vi "WS1050 Read From Configuration File.vi"(8 "error in (no error)":errorcluster, 11 "Configuration File Path":path=path "S:/Software_Control/RELEASED_SOFTWARE_RUN_ALL_TEST_FROM_HERE/PACKAGE/TMN/TMN1P5-Test-System/WS1050_vsa20-20_Temp.txt") -> (0 "error out":errorcluster, 3 "Configuration":T1)   [LabVIEW 2017]
uses:
  Andy's LLB LV2012/Read_Test_Limits/TSTR Configuration Cluster1.0.ctl
  <vilib>/Utility/config.llb/Read Key (String).vi
  <vilib>/Utility/config.llb/NI_LVConfig.lvlib
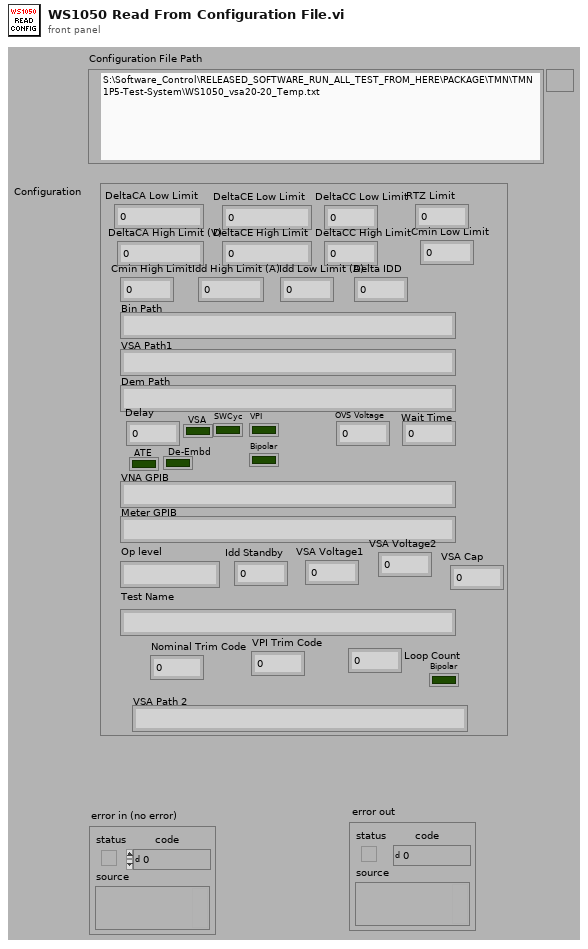
[diagram p1: front panel]
types:
  T1 = typedef "TSTR Configuration Cluster1.0.ctl" = cluster{"DeltaCA Low Limit ":dbl, "DeltaCA High Limit (V)":dbl, "DeltaCE Low Limit ":dbl, "DeltaCE High Limit":dbl, "DeltaCC Low Limit":dbl, "DeltaCC High Limit":dbl, "RTZ Limit":dbl, "Cmin Low Limit":dbl, "Cmin High Limit":dbl, "Idd High Limit (A)":dbl, "Idd Low Limit (A)":dbl, "Delta IDD":dbl, "Bin Path":string, "VSA Path1":string, "Dem Path":string, "Delay":dbl, "VSA":bool, "SWCyc":bool, "VPI":bool, "Bipolar":bool, "OVS Voltage":dbl, "Wait Time":dbl, "ATE":bool, "VNA GPIB":string, "Meter GPIB ":string, "Op level":string, "Idd Standby":dbl, "VSA Voltage1":dbl, "VSA Cap":dbl, "Test Name":string, "Nominal Trim Code":i32, "VPI Trim Code":i32, "De-Embd":bool, "Loop Count":i32, "Bipolar":bool, "VSA Path 2":string, "VSA Voltage2":dbl}
  T2 = typedef "NI_LVConfig.lvlib/Config Data RefNum.ctl" = refnum<k1>
  T3 = cluster{dbl, dbl, dbl, dbl, dbl, dbl, dbl, dbl, dbl, dbl, dbl, dbl, "value":string, "value":string, "value":string, dbl, bool, bool, bool, bool, dbl, dbl, bool, "value":string, "value":string, "value":string, dbl, dbl, dbl, "value":string, i32, i32, bool, i32, bool, "value":string, dbl}
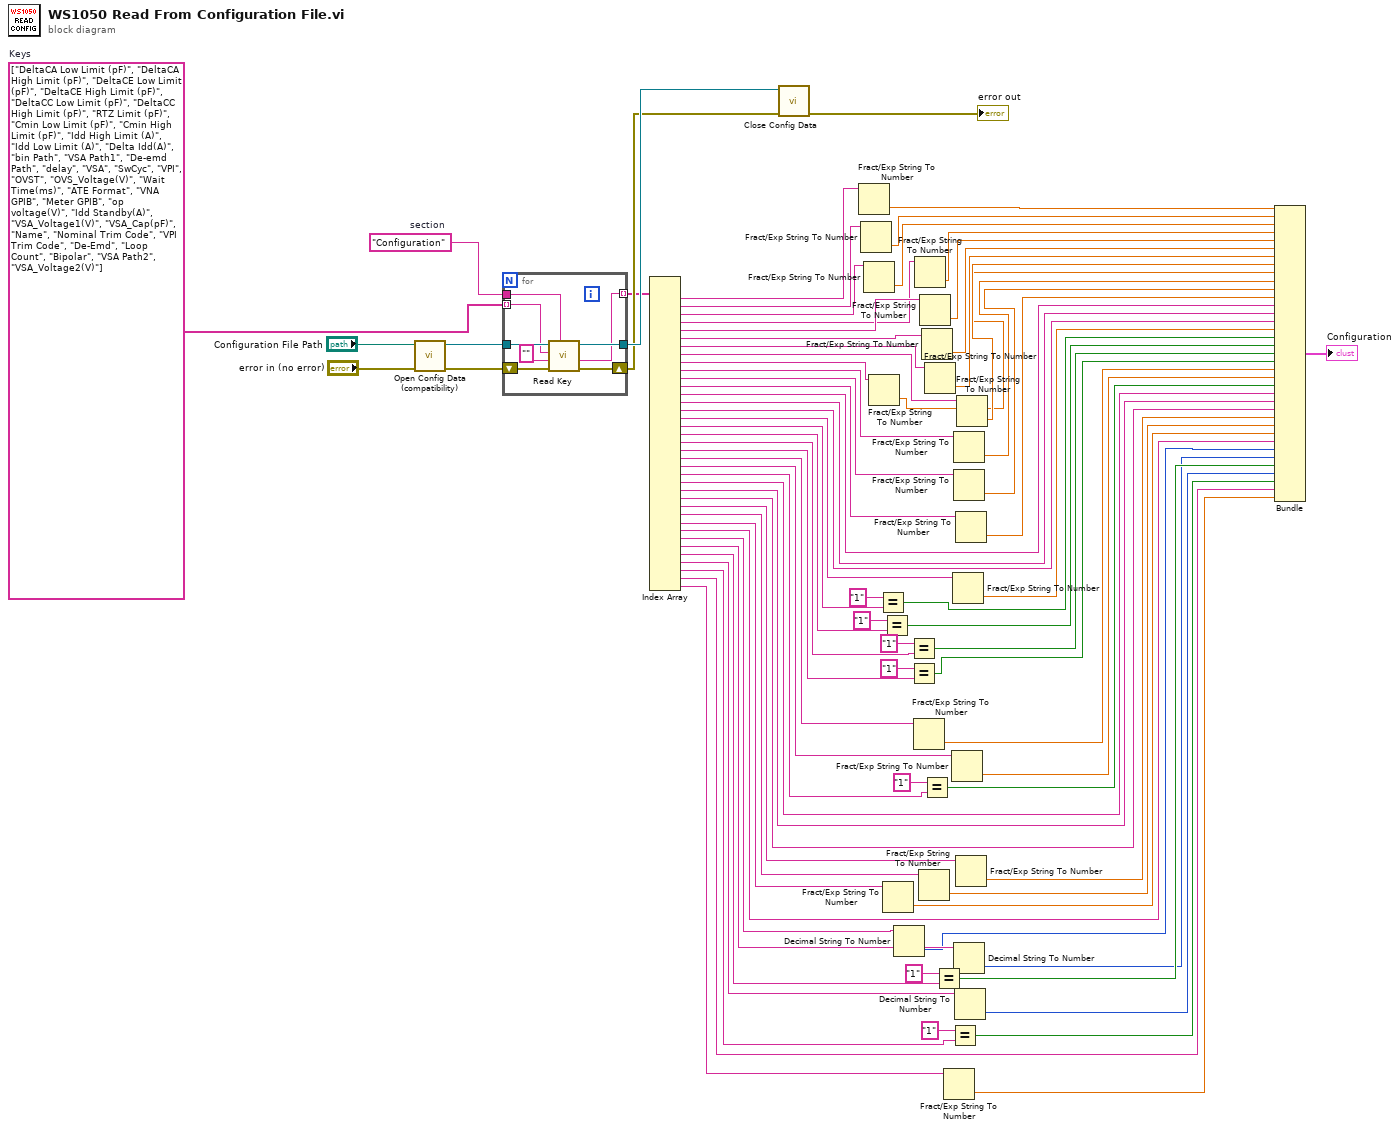
[diagram p0: block diagram]
diagram:
  w78 = string[] ["DeltaCA Low Limit (pF)", "DeltaCA High Limit (pF)", "DeltaCE Low Limit (pF)", "DeltaCE High Limit (pF)", "DeltaCC Low Limit (pF)", "DeltaCC High Limit (pF)", "RTZ Limit (pF)", "Cmin Low Limit (pF)", "Cmin High Limit (pF)", "Idd High Limit (A)", "Idd Low Limit (A)", "Delta Idd(A)", "bin Path", "VSA Path1", "De-emd Path", "delay", "VSA", "SwCyc", "VPI", "OVST", "OVS_Voltage(V)", "Wait Time(ms)", "ATE Format", "VNA GPIB", "Meter GPIB", "op voltage(V)", "Idd Standby(A)", "VSA_Voltage1(V)", "VSA_Cap(pF)", "Name", "Nominal Trim Code", "VPI Trim Code", "De-Emd", "Loop Count", "Bipolar", "VSA Path2", "VSA_Voltage2(V)"]  # Keys
  w79 = "Configuration"  # section
  n1 = call <vilib>:"Open Config Data (compatibility).vi"("error in (no error)"="error in (no error)", "configuration file path"="Configuration File Path") -> ("error out"=w82:errorcluster, "refnum"=w84:T2)  [unwired: 7 in, 1 out]
  n2 = for {
    tunnel: w84 -> [w92]
    tunnel: [w91] -> w83
    tunnel: w79 -> [w88]
    tunnel: [w87] -> w77 mode=indexing
    shift-right: [w89] -> w81
    shift-left: w82 -> [w90]
    tunnel: w78 -> [w86] mode=indexing
    n3 = call-poly <vilib>:"Read Key.vi"("section"=w88, "error in (no error)"=w90, "default value"="", "key"=w86, "refnum"=w92) -> ("error out"=w89:errorcluster, "value"=w87:string, "refnum out"=w91:T2)  [unwired: 1 in, 3 out]
  }
  n4 = Index Array(array=w77) -> (element #1=w75:string, element #2=w74:string, element #3=w68:string, element #4=w66:string, element #5=w73:string, element #6=w61:string, element #7=w60:string, element #8=w59:string, element #9=w58:string, element #10=w56:string, element #11=w53:string, element #12=w52:string, element #13=w50:string, element #14=w49:string, element #15=w48:string, element #16=w47:string, element #17=w45:string, element #18=w41:string, element #19=w38:string, element #20=w36:string, element #21=w29:string, element #22=w28:string, element #23=w27:string, element #24=w26:string, element #25=w25:string, element #26=w23:string, element #27=w24:string, element #28=w21:string, element #29=w20:string, element #30=w17:string, element #31=w16:string, element #32=w15:string, element #33=w12:string, element #34=w9:string, element #35=w6:string, element #36=w4:string, element #37=w3:string)  [unwired: 37 in]
  n5 = call <vilib>:"Close Config Data.vi"("error in (no error)"=w81, "refnum"=w83) -> ("error out"=→"error out":errorcluster)  [unwired: 1 in, 8 out]
  n6 = Fract/Exp String To Number(string=w75) -> (number=w72:dbl)  [unwired: 4 out]
  n7 = Fract/Exp String To Number(string=w74) -> (number=w69:dbl)  [unwired: 4 out]
  n8 = Fract/Exp String To Number(string=w68) -> (number=w67:dbl)  [unwired: 4 out]
  n9 = Fract/Exp String To Number(string=w58) -> (number=w57:dbl)  [unwired: 4 out]
  n10 = Equal?(x="1", y=w45) -> (x = y?=w43:bool)
  n11 = Equal?(x="1", y=w41) -> (x = y?=w40:bool)
  n12 = Fract/Exp String To Number(string=w20) -> (number=w18:dbl)  [unwired: 4 out]
  n13 = Decimal String To Number(string=w16) -> (number=w14:i32)  [unwired: 3 out]
  n14 = Equal?(x="1", y=w38) -> (x = y?=w37:bool)
  n15 = Equal?(x="1", y=w36) -> (x = y?=w35:bool)
  n16 = Fract/Exp String To Number(string=w29) -> (number=w32:dbl)  [unwired: 4 out]
  n17 = Fract/Exp String To Number(string=w66) -> (number=w65:dbl)  [unwired: 4 out]
  n18 = Fract/Exp String To Number(string=w21) -> (number=w19:dbl)  [unwired: 4 out]
  n19 = Fract/Exp String To Number(string=w73) -> (number=w71:dbl)  [unwired: 4 out]
  n20 = Fract/Exp String To Number(string=w61) -> (number=w64:dbl)  [unwired: 4 out]
  n21 = Equal?(x="1", y=w27) -> (x = y?=w30:bool)
  n22 = Fract/Exp String To Number(string=w60) -> (number=w63:dbl)  [unwired: 4 out]
  n23 = Equal?(x="1", y=w12) -> (x = y?=w11:bool)
  n24 = Fract/Exp String To Number(string=w3) -> (number=w2:dbl)  [unwired: 4 out]
  n25 = Equal?(x="1", y=w6) -> (x = y?=w5:bool)
  n26 = Fract/Exp String To Number(string=w28) -> (number=w31:dbl)  [unwired: 4 out]
  n27 = Fract/Exp String To Number(string=w47) -> (number=w46:dbl)  [unwired: 4 out]
  n28 = Fract/Exp String To Number(string=w56) -> (number=w55:dbl)  [unwired: 4 out]
  n29 = Fract/Exp String To Number(string=w53) -> (number=w54:dbl)  [unwired: 4 out]
  n30 = Decimal String To Number(string=w15) -> (number=w10:i32)  [unwired: 3 out]
  n31 = Decimal String To Number(string=w9) -> (number=w8:i32)  [unwired: 3 out]
  n32 = Fract/Exp String To Number(string=w52) -> (number=w51:dbl)  [unwired: 4 out]
  n33 = Fract/Exp String To Number(string=w24) -> (number=w22:dbl)  [unwired: 4 out]
  n34 = Fract/Exp String To Number(string=w59) -> (number=w62:dbl)  [unwired: 4 out]
  n35 = Bundle "Bundle"(w72, w69, w67, w65, w71, w64, w63, w62, w57, w55, w54, w51, "value"=w50, "value"=w49, "value"=w48, w46, w43, w40, w37, w35, w32, w31, w30, "value"=w26, "value"=w25, "value"=w23, w22, w19, w18, "value"=w17, w14, w10, w11, w8, w5, "value"=w4, w2) -> (→"Configuration":T3)  [unwired: 1 out]
